vi "Main.vi"() -> ()   [LabVIEW 2019]
doc: "Main VI for the InsightCM PortChecker application."
uses:
  controls/Ports to Check.ctl
  controls/States.ctl
  controls/Log Data Cluster.ctl
  controls/Communication Types.ctl
panel:
  in  "InsightCM Server Address":string="127.0.0.1"
  in  "User Panel":enum32{"User Panel"}(tab)
  in  "stop":bool
  in  "Edit Configuration":bool
  in  "Start Test":bool
  in  "View Results":bool
  in  "Log Results":bool
  out "current_tcp_port":u16
  in  "remote address":string="127.0.0.1"
  out "udp_port_under_test":u16
  out "Ports to Check":T1={"TCP Ports"=[82, 482, 5672, 6343, 8002, 49580, 3580, 80, 22, 44516, 52725, 8080], "UDP Ports"=[5353, 44515, 44525]}
  out "Connection Established?":bool
  out "UDP Received Array":dbl[](array[numeric])
  out "UDP Sent Array":dbl[](array[numeric])
  out "Current State":string
  out "error out":errorcluster
  out "Message from Server":string
  # "User Panel"
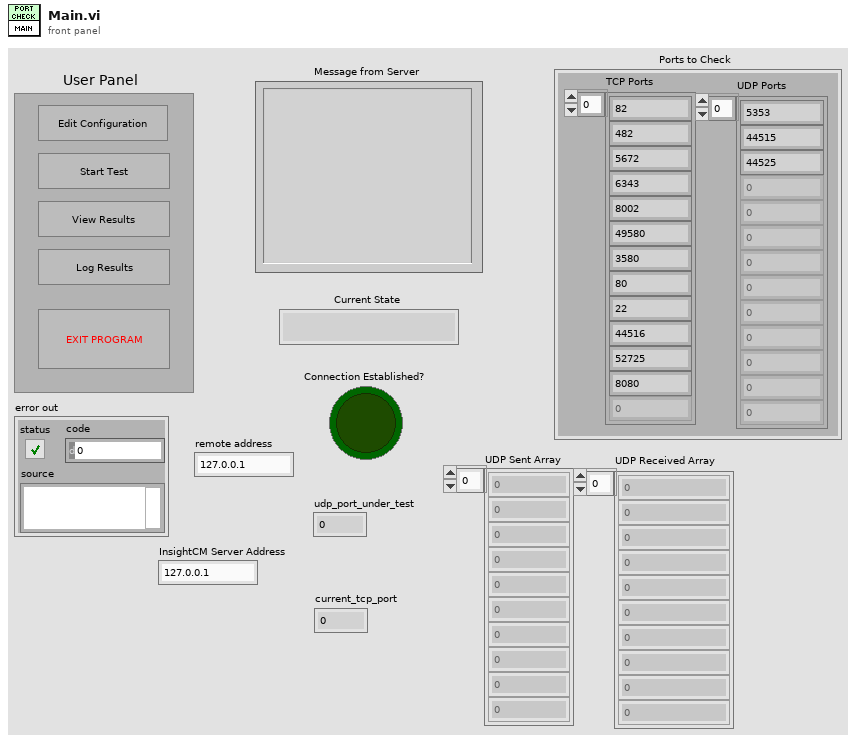
[diagram p1: front panel]
types:
  T1 = typedef "Ports to Check.ctl" = cluster{"TCP Ports":u32[], "UDP Ports":u32[]}
  T2 = typedef "States.ctl" = enum16{"Initialize", "Idle", "Edit Configuration", "Start Test", "TCP Tests", "UDP Tests", "View Results", "Test Complete", "Log Results", "Stop"}
  T3 = enum8{"Enabled", "Disabled", "Disabled and Grayed Out"}
  T4 = typedef "Communication Types.ctl" = enum16{"UDP - Server to Client", "UDP - Client to Server", "TCP - Server to Client", "TCP - Client to Server"}
  T5 = typedef "Log Data Cluster.ctl" = cluster{"Time Stamp":timestamp, "Port Number":u16, "Communication Type":T4, "success?":bool, "error in":errorcluster}
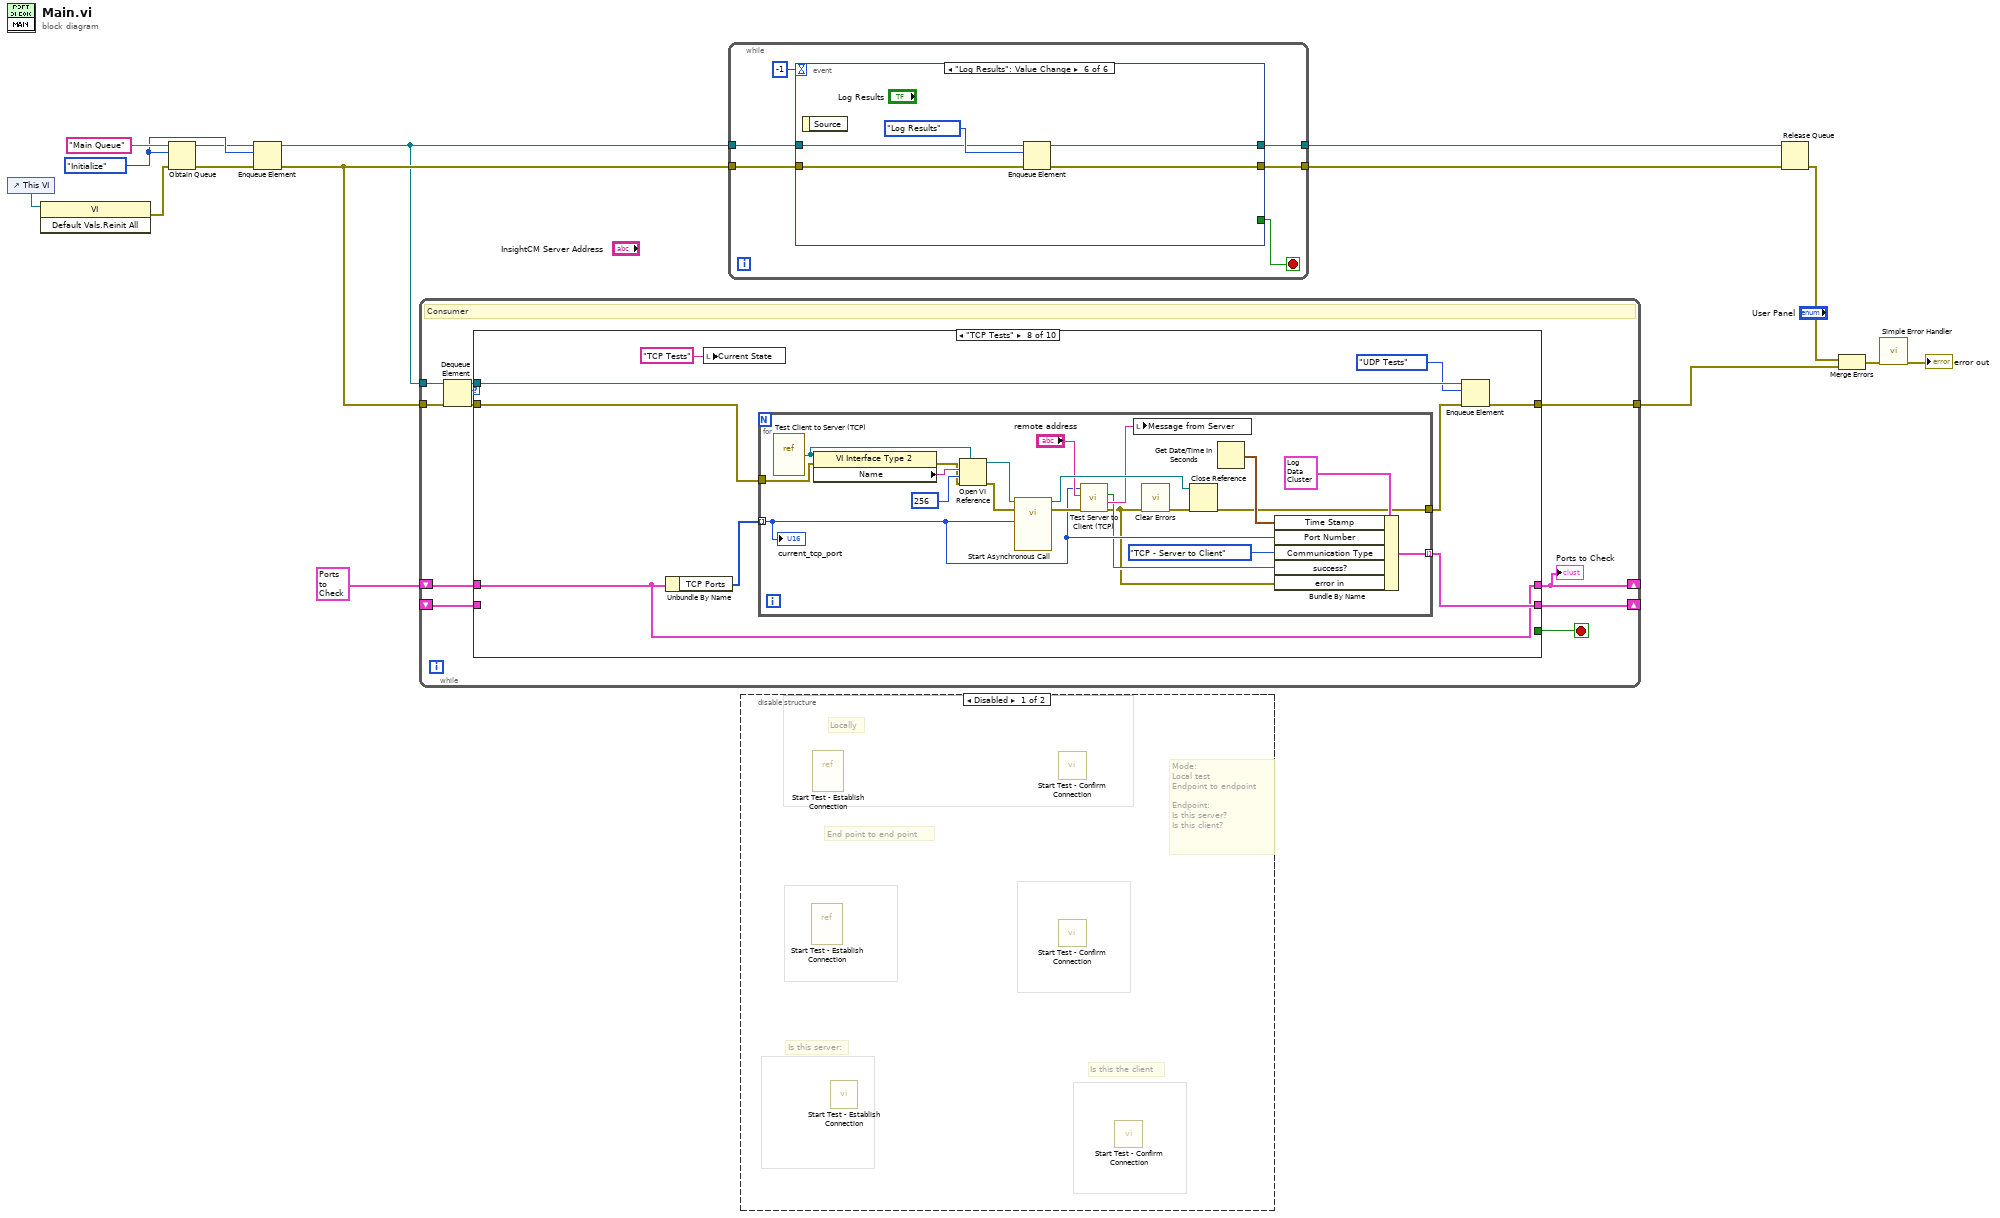
[diagram p0: block diagram]
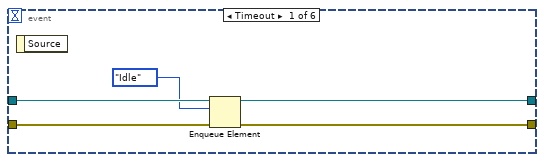
[diagram p3: hidden frame]
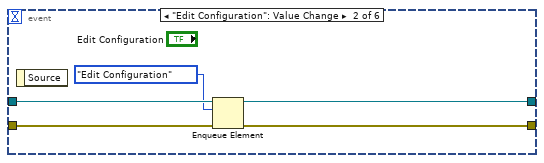
[diagram p4: hidden frame]
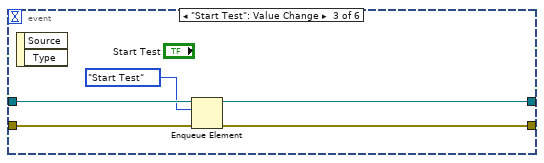
[diagram p5: hidden frame]
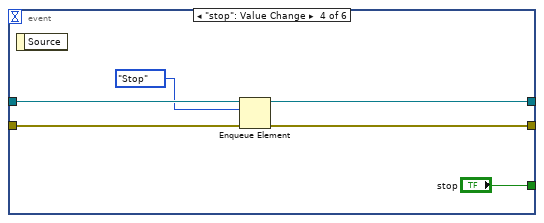
[diagram p6: hidden frame]
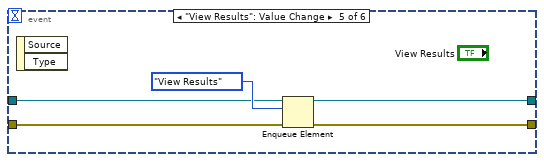
[diagram p7: hidden frame]
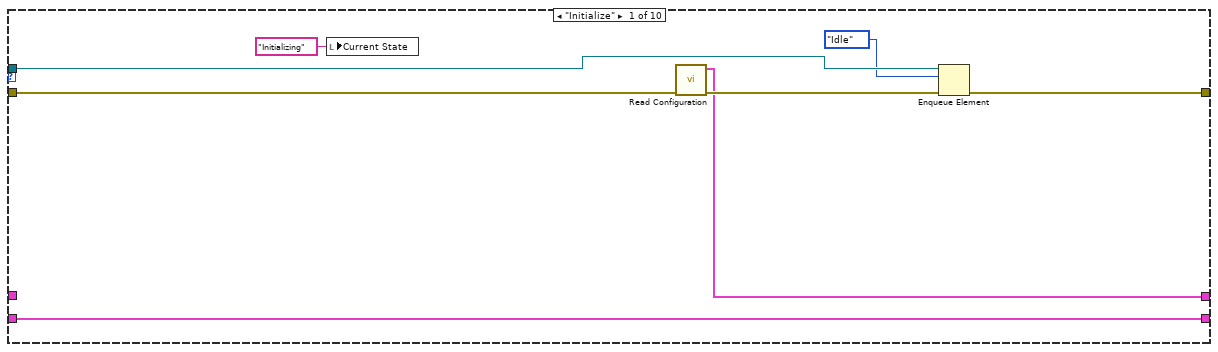
[diagram p8: hidden frame]
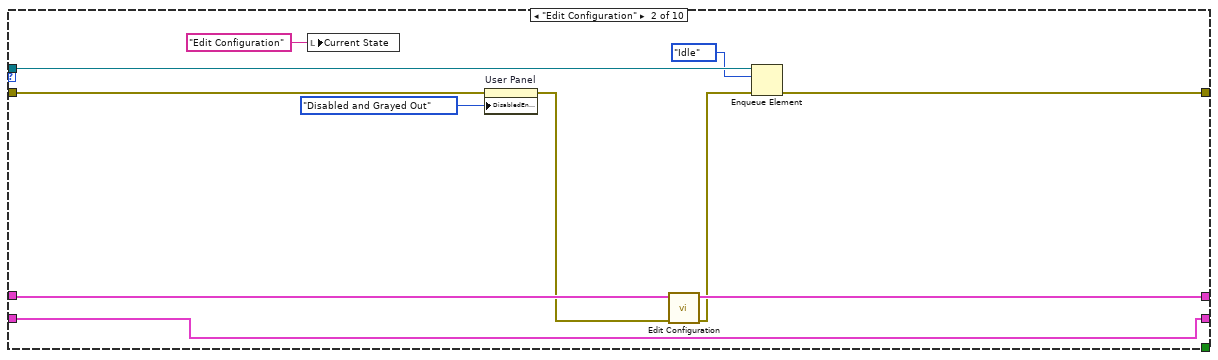
[diagram p9: hidden frame]
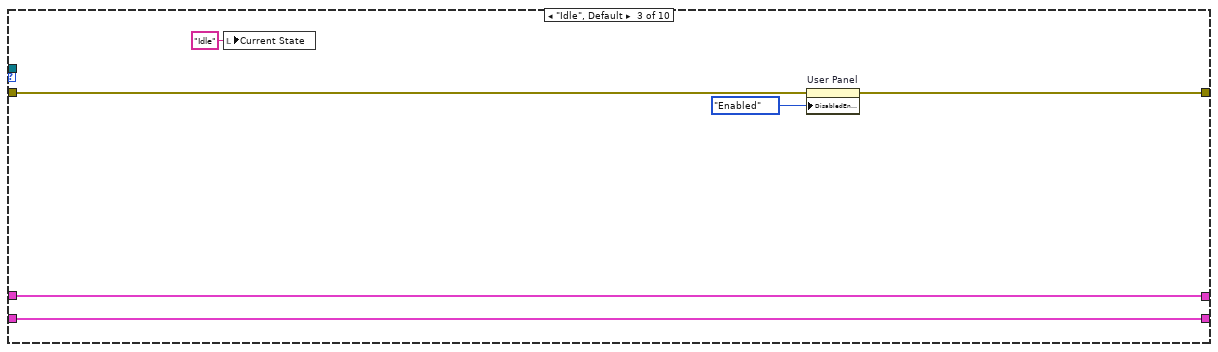
[diagram p10: hidden frame]
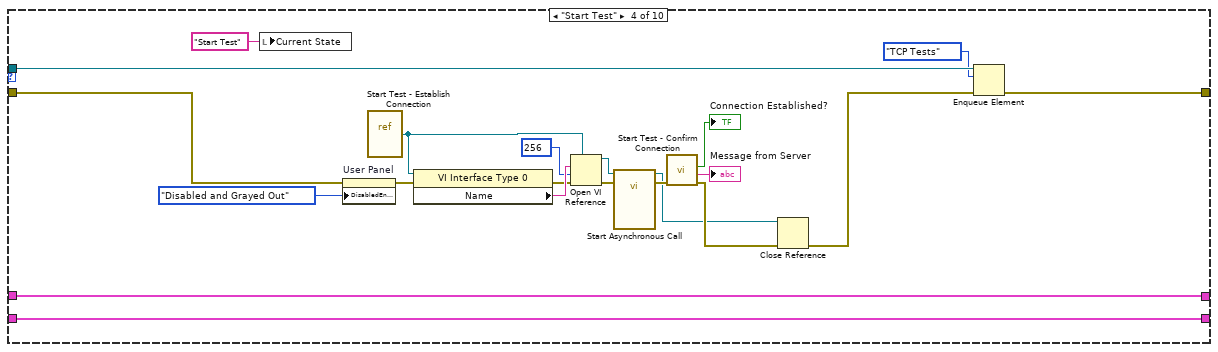
[diagram p11: hidden frame]
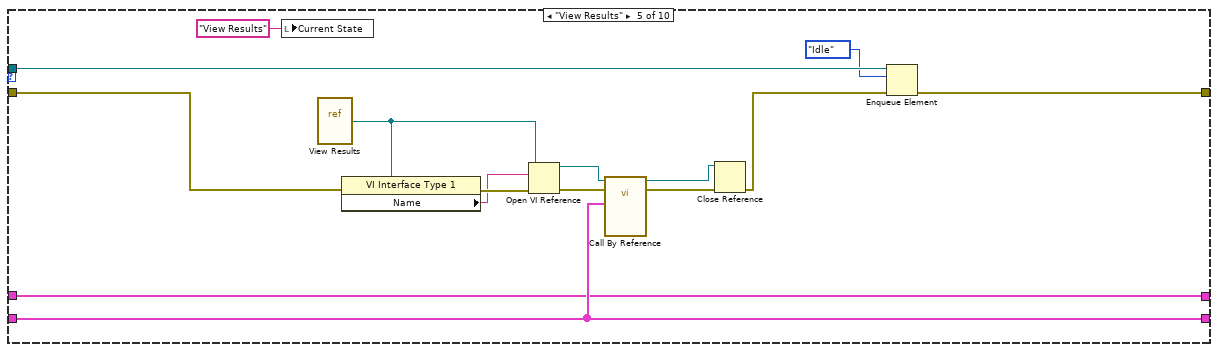
[diagram p12: hidden frame]
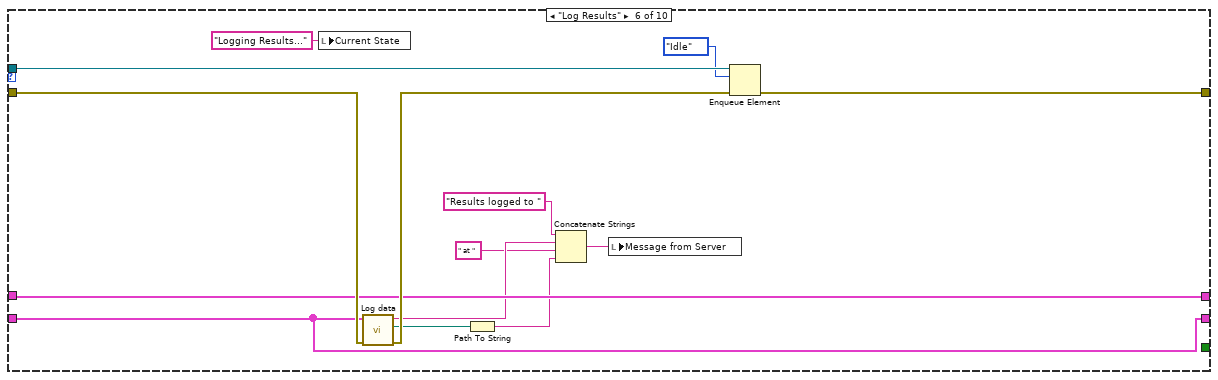
[diagram p13: hidden frame]
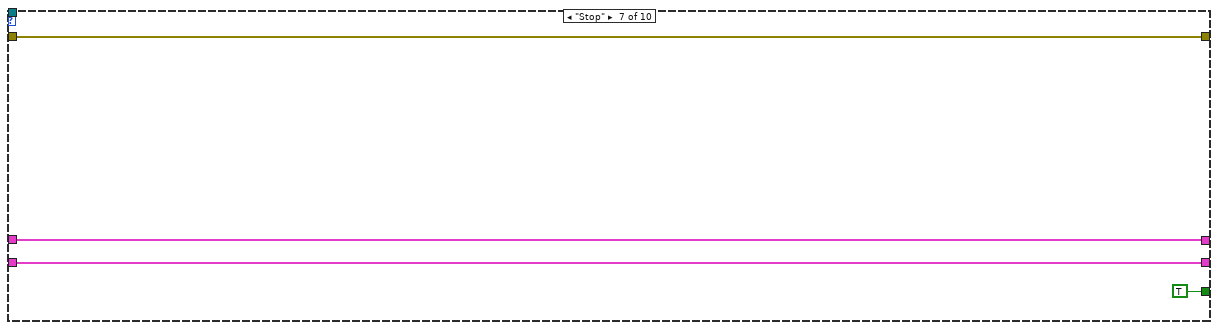
[diagram p14: hidden frame]
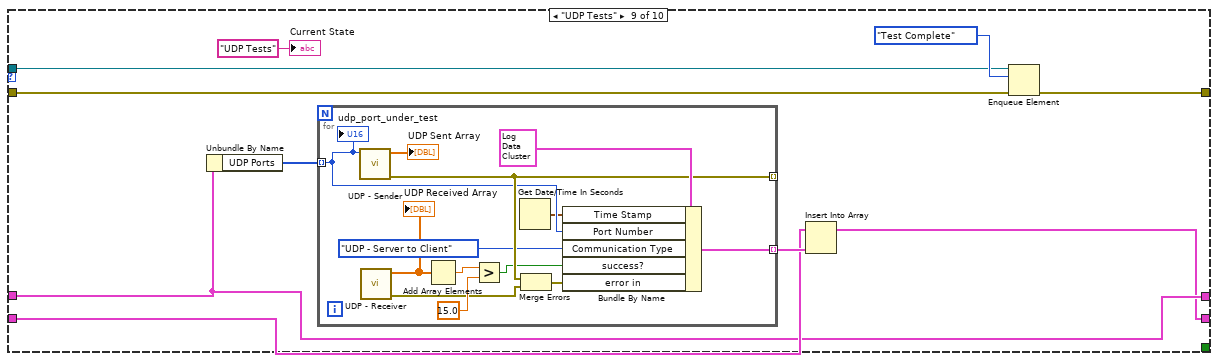
[diagram p15: hidden frame]
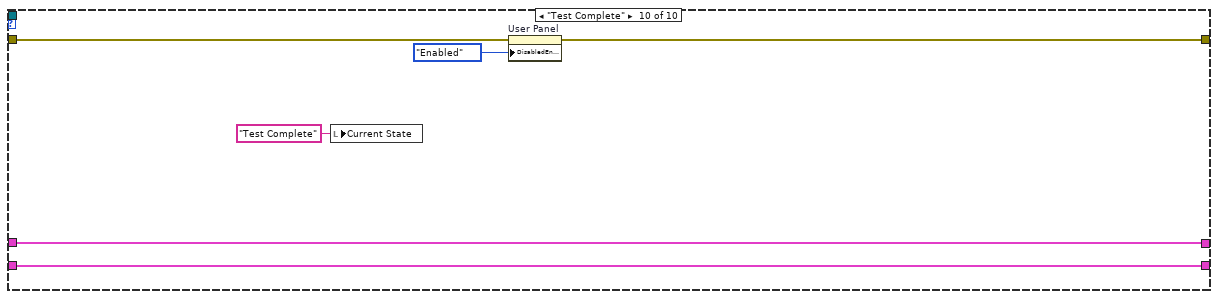
[diagram p16: hidden frame]
diagram:
  w5 = States."Initialize" ("States")
  n1 = control-ref of="This VI"() -> (w8:refnum<vi>)
  n2 = invoke class="VI" method="Default Vals.Reinit All"(reference=w8) -> (error out=w7:errorcluster)  [unwired: 2 in, 2 out]
  n3 = Obtain Queue(name (unnamed)="Main Queue", element data type=w5, error in (no error)=w7) -> (queue out=w3:refnum<queue>, error out=w9:errorcluster)  [unwired: 2 in, 1 out]
  n4 = Enqueue Element(queue=w3, element=w5, error in (no error)=w9) -> (queue out=w4:refnum<queue>, error out=w6:errorcluster)  [unwired: 1 in, 1 out]
  n5 = while {
    tunnel: w4 -> [w26]
    tunnel: w6 -> [w23]
    tunnel: [w21] -> w1
    shift-right: [w18] -> _
    shift-left: _ -> [w17]
    shift-right: [w16] -> _
    shift-left: T1 {"TCP Ports"=[82, 482, 5672, 6343, 8002, 49580, 3580, 80, 22, 44516, 52725, 8080], "UDP Ports"=[5353, 44515, 44525]} ("Ports to Check") -> [w19]
    stop <- w24 stop-if-true
    # "Consumer"
    n6 = Dequeue Element(queue=w26, error in (no error)=w23) -> (queue out=w20:refnum<queue>, element=w25:T2, error out=w22:errorcluster)  [unwired: 1 in, 1 out]
    n7 = case shown="\"TCP Tests\"" w25 {
      tunnel: [_ _ _ _ _ _ TRUE _ _ _] -> w24
      tunnel: w22 -> [w34 w36 w47 w53 w79 w100 w104 w109 w143 w159]
      tunnel: [w30 w41 w46 w71 w78 w97 w104 w111 w141 w158] -> w21
      tunnel: w20 -> [w29 w40 _ w66 w77 w98 _ w114 w142 _]
      tunnel: w19 -> [_ w44 w50 w57 w80 w95 w103 w106 w136 w162]
      tunnel: [w27 w38 w49 w56 w86 w88 w102 w107 w135 w161] -> w18
      tunnel: w17 -> [w27 w38 w49 w56 w86 w88 w102 _ w137 w161]
      tunnel: [w32 w43 w50 w57 w80 w95 w103 w106 w136 w162] -> w16
      frame "Initialize" {
        n8 = local write "Current State"("Initializing" ("Current State")) -> ()
        n9 = call "Read Configuration.vi"("error in (no error)"=w34) -> ("error out"=w33:errorcluster, "Ports to Check"=w32:T1)  [unwired: 9 in]
        n10 = Enqueue Element(queue=w29, element=States."Idle" ("States"), error in (no error)=w33) -> (error out=w30:errorcluster)  [unwired: 1 in, 2 out]
      }
      frame "Edit Configuration" {
        n11 = local write "Current State"("Edit Configuration" ("message")) -> ()
        n12 = property on="User Panel" class="TabCtl (strict)"(error in=w36, "DisabledEnum"=T3."Disabled and Grayed Out" ("Disabled")) -> (error out=w35:errorcluster)  [unwired: 1 in, 1 out]
        n13 = call "Edit Configuration.vi"("error in (no error)"=w35, "Ports to Check"=w44) -> ("error out"=w42:errorcluster, "Ports to Check"=w43:T1)  [unwired: 8 in]
        n14 = Enqueue Element(queue=w40, element=States."Idle", error in (no error)=w42) -> (error out=w41:errorcluster)  [unwired: 1 in, 2 out]
      }
      frame "Idle", Default {
        n15 = local write "Current State"("Idle" ("Current State")) -> ()
        n16 = property on="User Panel" class="TabCtl (strict)"(error in=w47, "DisabledEnum"=T3."Enabled" ("Disabled")) -> (error out=w46:errorcluster)  [unwired: 1 in, 1 out]
      }
      frame "Start Test" {
        n17 = local write "Current State"("Start Test" ("message")) -> ()
        n18 = property on="User Panel" class="TabCtl (strict)"(error in=w53, "DisabledEnum"=T3."Disabled and Grayed Out" ("Disabled")) -> (error out=w54:errorcluster)  [unwired: 1 in, 1 out]
        n19 = vi-ref "Start Test - Establish Connection.vi"() -> (w63:refnum<vi>)
        n20 = property class="VI Interface Type 0"(reference=w63, error in=w54) -> (error out=w64:errorcluster, "Name"=w65:string)  [unwired: 1 out]
        n21 = Open VI Reference(type specifier VI Refnum (for type only)=w63, vi path=w65, options=256, error in (no error)=w64) -> (vi reference=w70:refnum<vi>, error out=w69:errorcluster)  [unwired: 2 in]
        n22 = call-by-ref "Start Asynchronous Call"(reference=w70, error in=w69) -> (reference out=w52:refnum<vi>, error out=w72:errorcluster)  [unwired: 10 in, 1 out]
        n23 = call "Start Test - Confirm Connection.vi"("error in (no error)"=w72) -> ("Connection Established"=→"Connection Established?":bool, "Message from Server"=→"Message from Server":string, "error out"=w68:errorcluster)  [unwired: 7 in]
        n24 = Close Reference(reference=w52, error in (no error)=w68) -> (error out=w67:errorcluster)
        n25 = Enqueue Element(queue=w66, element=States."TCP Tests" ("States"), error in (no error)=w67) -> (error out=w71:errorcluster)  [unwired: 1 in, 2 out]
      }
      frame "View Results" {
        n26 = local write "Current State"("View Results" ("message")) -> ()
        n27 = vi-ref "View Results.vi"() -> (w83:refnum<vi>)
        n28 = property class="VI Interface Type 1"(reference=w83, error in=w79) -> (error out=w82:errorcluster, "Name"=w81:string)  [unwired: 1 out]
        n29 = Open VI Reference(type specifier VI Refnum (for type only)=w83, vi path=w81, error in (no error)=w82) -> (vi reference=w84:refnum<vi>, error out=w85:errorcluster)  [unwired: 3 in]
        n30 = call-by-ref "?"(reference=w84, error in=w85, "Results"=w86) -> (reference out=w73:refnum<vi>, error out=w75:errorcluster)  [unwired: 10 in, 1 out]
        n31 = Close Reference(reference=w73, error in (no error)=w75) -> (error out=w74:errorcluster)
        n32 = Enqueue Element(queue=w77, element=States."Idle", error in (no error)=w74) -> (error out=w78:errorcluster)  [unwired: 1 in, 2 out]
      }
      frame "Log Results" {
        n33 = local write "Current State"("Logging Results..." ("message")) -> ()
        n34 = call "Log data.vi"("error in (no error)"=w100, "Results"=w88) -> ("error out"=w99:errorcluster, "log file path"=w90:path, "log file name"=w93:string)  [unwired: 7 in]
        n35 = Path To String(path=w90) -> (string=w89:string)
        n36 = Concatenate Strings("Results logged to " ("Message from Server"), w93, " at " ("string"), w89) -> (w92:string)
        n37 = local write "Message from Server"(w92) -> ()
        n38 = Enqueue Element(queue=w98, element=States."Idle" ("States"), error in (no error)=w99) -> (error out=w97:errorcluster)  [unwired: 1 in, 2 out]
      }
      frame "Stop" {
      }
      frame "TCP Tests" {
        n39 = Unbundle By Name(w106) -> ("TCP Ports"=w110:u32[])
        n40 = local write "Current State"("TCP Tests" ("message")) -> ()
        n41 = for {
          tunnel: w110 -> [w122] mode=indexing
          tunnel: [w119] -> w108
          tunnel: w109 -> [w128]
          tunnel: [w118] -> w107 mode=indexing
          n42 = vi-ref "Test Client to Server (TCP).vi"() -> (w133:refnum<vi>)
          n43 = property class="VI Interface Type 2"(reference=w133, error in=w128) -> (error out=w127:errorcluster, "Name"=w132:string)  [unwired: 1 out]
          n44 = Open VI Reference(type specifier VI Refnum (for type only)=w133, vi path=w132, options=256, error in (no error)=w127) -> (vi reference=w131:refnum<vi>, error out=w126:errorcluster)  [unwired: 2 in]
          n45 = call-by-ref "Start Asynchronous Call"(reference=w131, error in=w126, "port"=w122) -> (reference out=w129:refnum<vi>, error out=w130:errorcluster)  [unwired: 7 in, 3 out]
          n46 = call "Test Server to Client (TCP).vi"("remote port or service name"=w122, "address"="remote address", "error in (no error)"=w130) -> ("Connection Established"=w120:bool, "Message from Server"=w125:string, "error out"=w116:errorcluster)  [unwired: 5 in]
          n47 = local write "Message from Server"(w125) -> ()
          n48 = call <vilib>:"Clear Errors.vi"("error in (no error)"=w116) -> ("error out"=w115:errorcluster)  [unwired: 5 in, 1 out]
          n49 = Close Reference(reference=w129, error in (no error)=w115) -> (error out=w119:errorcluster)
          n50 = Get Date/Time In Seconds() -> (seconds since 1Jan1904=w121:timestamp)
          n51 = Bundle By Name(cluster=T5 {"Time Stamp"=timestamp(0 s since 1904-01-01), "Port Number"=0, "Communication Type"=enum."UDP - Server to Client", "success?"=FALSE, "error in"={"status"=FALSE, "code"=0, "source"=""}} ("log_data"), "Time Stamp"=w121, "Port Number"=w122, "Communication Type"=Communication_Types."TCP - Server to Client", "success?"=w120, "error in"=w116) -> (w118:T5)
          "current_tcp_port" <- w122
        }
        n52 = Enqueue Element(queue=w114, element=States."UDP Tests" ("States"), error in (no error)=w108) -> (error out=w111:errorcluster)  [unwired: 1 in, 2 out]
      }
      frame "UDP Tests" {
        n53 = Unbundle By Name(w136) -> ("UDP Ports"=w140:u32[])
        n54 = for {
          tunnel: w140 -> [w147] mode=indexing
          tunnel: [w151] -> _ mode=indexing
          tunnel: [w145] -> w138 mode=indexing
          n55 = call "UDP - Sender.vi"("port"=w147) -> ("error out"=w151:errorcluster, "Array Out"=→"UDP Sent Array":dbl[])  [unwired: 8 in, 1 out]
          n56 = call "UDP - Receiver.vi"() -> ("error out"=w150:errorcluster, "UDP Received Array"=w156:dbl[])  [unwired: 9 in, 1 out]
          "UDP Received Array" <- w156
          n57 = Add Array Elements(numeric array=w156) -> (sum=w155:dbl)
          n58 = Greater?(x=w155, y=15.0) -> (0:w149:bool)
          n59 = Get Date/Time In Seconds() -> (seconds since 1Jan1904=w146:timestamp)
          n60 = Merge Errors(w151, w150) -> (w152:errorcluster)
          n61 = Bundle By Name(cluster=T5 {"Time Stamp"=timestamp(0 s since 1904-01-01), "Port Number"=0, "Communication Type"=enum."UDP - Server to Client", "success?"=FALSE, "error in"={"status"=FALSE, "code"=0, "source"=""}} ("log_data"), "Time Stamp"=w146, "Port Number"=w147, "Communication Type"=Communication_Types."UDP - Server to Client", "success?"=w149, "error in"=w152) -> (w145:T5)
          "udp_port_under_test" <- w147
        }
        n62 = Insert Into Array(array=w137, new element=w138) -> (w135:T5[])  [unwired: 1 in]
        n63 = Enqueue Element(queue=w142, element=States."Test Complete" ("States"), error in (no error)=w143) -> (error out=w141:errorcluster)  [unwired: 1 in, 2 out]
        "Current State" <- "UDP Tests" ("message")
      }
      frame "Test Complete" {
        n64 = local write "Current State"("Test Complete" ("Current State")) -> ()
        n65 = property on="User Panel" class="TabCtl (strict)"(error in=w159, "DisabledEnum"=T3."Enabled" ("Disabled")) -> (error out=w158:errorcluster)  [unwired: 1 in, 1 out]
      }
    }
    "Ports to Check" <- w16
  }
  n66 = while {
    tunnel: w4 -> [w169]
    tunnel: [w168] -> w14
    tunnel: w6 -> [w166]
    tunnel: [w165] -> w11
    stop <- w167 stop-if-true
    n67 = event shown="[5] \"Log Results\": Value Change" {
      selector: _ -> [_ _ _ _ _ _]
      dyn-events: _ -> [_ _ _ _ _ _]
      timeout: -1 -> [_ _ _ _ _ _]
      tunnel: w169 -> [w174 w179 w184 w189 w194 w199]
      tunnel: [w173 w177 w182 w188 w193 w198] -> w168
      tunnel: [_ _ _ "stop" _ _] -> w167
      tunnel: w166 -> [w172 w176 w181 w186 w192 w197]
      tunnel: [w171 w175 w180 w185 w191 w196] -> w165
      event Timeout {
        n68 = event-data() -> ()  [unwired: 1 in, 1 out]
        n69 = Enqueue Element(queue=w174, element=States."Idle" ("States"), error in (no error)=w172) -> (queue out=w173:refnum<queue>, error out=w171:errorcluster)  [unwired: 1 in, 1 out]
      }
      event "Edit Configuration": Value Change {
        n70 = event-data() -> ()  [unwired: 1 in, 1 out]
        n71 = Enqueue Element(queue=w179, element=States."Edit Configuration" ("States"), error in (no error)=w176) -> (queue out=w177:refnum<queue>, error out=w175:errorcluster)  [unwired: 1 in, 1 out]
      }
      event "Start Test": Value Change {
        n72 = event-data() -> ()  [unwired: 1 in, 2 out]
        n73 = Enqueue Element(queue=w184, element=States."Start Test" ("States"), error in (no error)=w181) -> (queue out=w182:refnum<queue>, error out=w180:errorcluster)  [unwired: 1 in, 1 out]
      }
      event "stop": Value Change {
        n74 = event-data() -> ()  [unwired: 1 in, 1 out]
        n75 = Enqueue Element(queue=w189, element=States."Stop" ("States"), error in (no error)=w186) -> (queue out=w188:refnum<queue>, error out=w185:errorcluster)  [unwired: 1 in, 1 out]
      }
      event "View Results": Value Change {
        n76 = event-data() -> ()  [unwired: 1 in, 2 out]
        n77 = Enqueue Element(queue=w194, element=States."View Results" ("States"), error in (no error)=w192) -> (queue out=w193:refnum<queue>, error out=w191:errorcluster)  [unwired: 1 in, 1 out]
      }
      event "Log Results": Value Change {
        n78 = event-data() -> ()  [unwired: 1 in, 1 out]
        n79 = Enqueue Element(queue=w199, element=States."Log Results" ("States"), error in (no error)=w197) -> (queue out=w198:refnum<queue>, error out=w196:errorcluster)  [unwired: 1 in, 1 out]
      }
    }
  }
  n80 = disable-structure shown="Disabled" {
    frame Disabled {
      # "Is this the client"
      # "Is this server:"
      # "Mode:\nLocal test\nEndpoint to endpoint\n\nEndpoint:\nIs this server?\nIs this client?"
      # "End point to end point"
      # "Locally"
      n81 = vi-ref "Start Test - Establish Connection.vi"() -> ()  [unwired: 1 out]
      n82 = vi-ref "Start Test - Establish Connection.vi"() -> ()  [unwired: 1 out]
      n83 = call "Start Test - Establish Connection.vi"() -> ()  [unwired: 10 in, 1 out]
      n84 = call "Start Test - Confirm Connection.vi"() -> ()  [unwired: 8 in, 3 out]
      n85 = call "Start Test - Confirm Connection.vi"() -> ()  [unwired: 8 in, 3 out]
      n86 = call "Start Test - Confirm Connection.vi"() -> ()  [unwired: 8 in, 3 out]
    }
    frame Enabled {
    }
  }
  n87 = Release Queue(queue=w14, error in (no error)=w11) -> (error out=w10:errorcluster)  [unwired: 1 in, 2 out]
  n88 = Merge Errors(w10, w1) -> (w12:errorcluster)
  n89 = call <vilib>:"Simple Error Handler.vi"("error in (no error)"=w12) -> ("error out"=→"error out":errorcluster)  [unwired: 4 in, 4 out]
